vi "LED matrix.vi"() -> ()   [LabVIEW 2010]
uses:
  <vilib>/MakerHub/LINX/LMH-LINX.lvlib
  <vilib>/MakerHub/LINX/Private/Type Defs/Peripherals/SPI/SPI CS Logic Level.ctl
  <vilib>/MakerHub/LINX/Public/Peripherals/SPI/SPI CS Config.ctl
  <vilib>/MakerHub/LINX/Public/Peripherals/SPI/SPI Write Read N Frames.vi
  <vilib>/MakerHub/LINX/Private/Type Defs/Peripherals/SPI/SPI Bit Order.ctl
  <vilib>/MakerHub/LINX/Private/Type Defs/Peripherals/SPI/SPI Mode.ctl
  <vilib>/MakerHub/LINX/Private/Type Defs/Peripherals/SPI/SPI Configuration.ctl
  <vilib>/MakerHub/LINX/Public/Utilities/Open Serial.vi
panel:
  out "Title":string="LabVIEW Arduino and LED matrix"
  in  "4":bool[][](array[boolean])=[[TRUE, TRUE, TRUE, TRUE, TRUE, TRUE, TRUE, TRUE], [TRUE, FALSE, FALSE, FALSE, FALSE, FALSE, FALSE, TRUE], [TRUE, FALSE, FALSE, FALSE, FALSE, FALSE, FALSE, TRUE], [TRUE, FALSE, FALSE, FALSE, FALSE, FALSE, FALSE, TRUE], [TRUE, FALSE, FALSE, FALSE, FALSE, FALSE, FALSE, TRUE], [TRUE, FALSE, FALSE, FALSE, FALSE, FALSE, FALSE, TRUE], [TRUE, FALSE, FALSE, FALSE, FALSE, FALSE, FALSE, TRUE], [TRUE, TRUE, TRUE, TRUE, TRUE, TRUE, TRUE, TRUE]]
  in  "milliseconds to wait":u32=1000
  in  "Debug":bool
  in  "1":bool[][](array[boolean])=[[FALSE, FALSE, FALSE, FALSE, FALSE, FALSE, FALSE, FALSE], [FALSE, FALSE, FALSE, FALSE, FALSE, FALSE, FALSE, FALSE], [FALSE, FALSE, FALSE, FALSE, FALSE, FALSE, FALSE, FALSE], [FALSE, FALSE, FALSE, TRUE, TRUE, FALSE, FALSE, FALSE], [FALSE, FALSE, FALSE, TRUE, TRUE, FALSE, FALSE, FALSE], [FALSE, FALSE, FALSE, FALSE, FALSE, FALSE, FALSE, FALSE], [FALSE, FALSE, FALSE, FALSE, FALSE, FALSE, FALSE, FALSE], [FALSE, FALSE, FALSE, FALSE, FALSE, FALSE, FALSE, FALSE]]
  in  "2":bool[][](array[boolean])=[[FALSE, FALSE, FALSE, FALSE, FALSE, FALSE, FALSE, FALSE], [FALSE, FALSE, FALSE, FALSE, FALSE, FALSE, FALSE, FALSE], [FALSE, FALSE, TRUE, TRUE, TRUE, TRUE, FALSE, FALSE], [FALSE, FALSE, TRUE, FALSE, FALSE, TRUE, FALSE, FALSE], [FALSE, FALSE, TRUE, FALSE, FALSE, TRUE, FALSE, FALSE], [FALSE, FALSE, TRUE, TRUE, TRUE, TRUE, FALSE, FALSE], [FALSE, FALSE, FALSE, FALSE, FALSE, FALSE, FALSE, FALSE], [FALSE, FALSE, FALSE, FALSE, FALSE, FALSE, FALSE, FALSE]]
  in  "3":bool[][](array[boolean])=[[FALSE, FALSE, FALSE, FALSE, FALSE, FALSE, FALSE, FALSE], [FALSE, TRUE, TRUE, TRUE, TRUE, TRUE, TRUE, FALSE], [FALSE, TRUE, FALSE, FALSE, FALSE, FALSE, TRUE, FALSE], [FALSE, TRUE, FALSE, FALSE, FALSE, FALSE, TRUE, FALSE], [FALSE, TRUE, FALSE, FALSE, FALSE, FALSE, TRUE, FALSE], [FALSE, TRUE, FALSE, FALSE, FALSE, FALSE, TRUE, FALSE], [FALSE, TRUE, TRUE, TRUE, TRUE, TRUE, TRUE, FALSE], [FALSE, FALSE, FALSE, FALSE, FALSE, FALSE, FALSE, FALSE]]
  out "Loop":i32=8
  in  "Serial Port":refnum<visa-resource-name>="COM4"
  in  "SPI Frame Size":u8=2
  in  "SPI Channel (0)":u8
  in  "stop":bool
  # "Ricky"
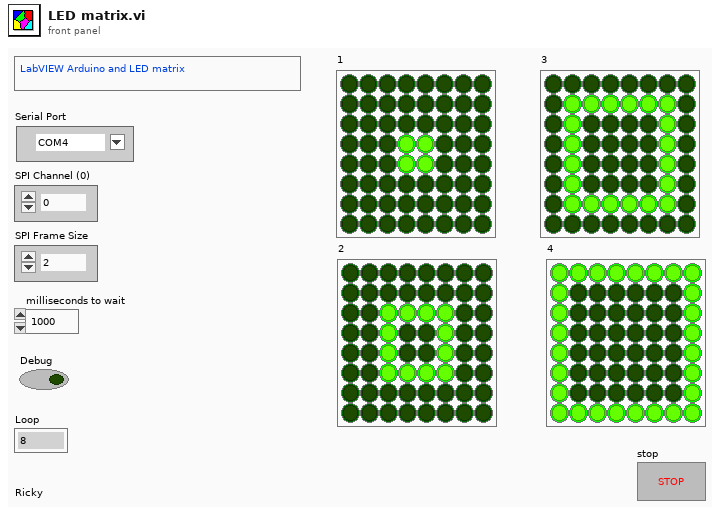
[diagram p1: front panel]
types:
  T1 = typedef "LMH-LINX.lvlib/SPI Configuration.ctl" = cluster{"Clock Frequency":u32, "Bit Order":T2, "SPI Mode":T3}
  T2 = typedef "LMH-LINX.lvlib/SPI Bit Order.ctl" = enum8{"LSb First", "MSb First"}
  T3 = typedef "LMH-LINX.lvlib/SPI Mode.ctl" = enum8{"Mode 0", "Mode 1", "Mode 2", "Mode 3"}
  T4 = typedef "LMH-LINX.lvlib/SPI CS Config.ctl" = cluster{"CS Channel":u8, "CS Logic Level":T5}
  T5 = typedef "LMH-LINX.lvlib/SPI CS Logic Level.ctl" = enum8{"Active Low", "Active High"}
  T6 = typedef "LMH-LINX.lvlib/LINX Ref.ctl" = cluster{"IO":T7, "Interface":T8, "LINX Device Config":T9}
  T7 = typedef "LMH-LINX.lvlib/Platform.ctl" = enum16{"Remote", "Local"}
  T8 = typedef "LMH-LINX.lvlib/Interface.ctl" = enum16{"Serial", "TCP"}
  T9 = typedef "LMH-LINX.lvlib/Device.lvlib/LINX Device Config.ctl" = cluster{"Interface":T8, "COM Port":refnum<visa-resource-name>, "TCP Configuration":T10, "Device Family":u8, "Device ID":u8, "Device Name":string, "TCP Ref":refnum<k5>, "Channels":T11}
  T10 = typedef "LMH-LINX.lvlib/Device.lvlib/TCP Config.ctl" = cluster{"IP Address":string, "Port":u16}
  T11 = typedef "LMH-LINX.lvlib/Channels.ctl" = cluster{"DI":u8[], "DO":u8[], "AI":u8[], "AO":u8[], "PWM":u8[], "QE":u8[], "UART":u8[], "I2C 2":u8[], "SPI":u8[], "CAN":u8[], "Servo":u8[], "AI Ref (V)":dbl, "AI Resolution (Bits)":u8, "AO Ref (V)":dbl, "AO Resolution (Bits)":u8}
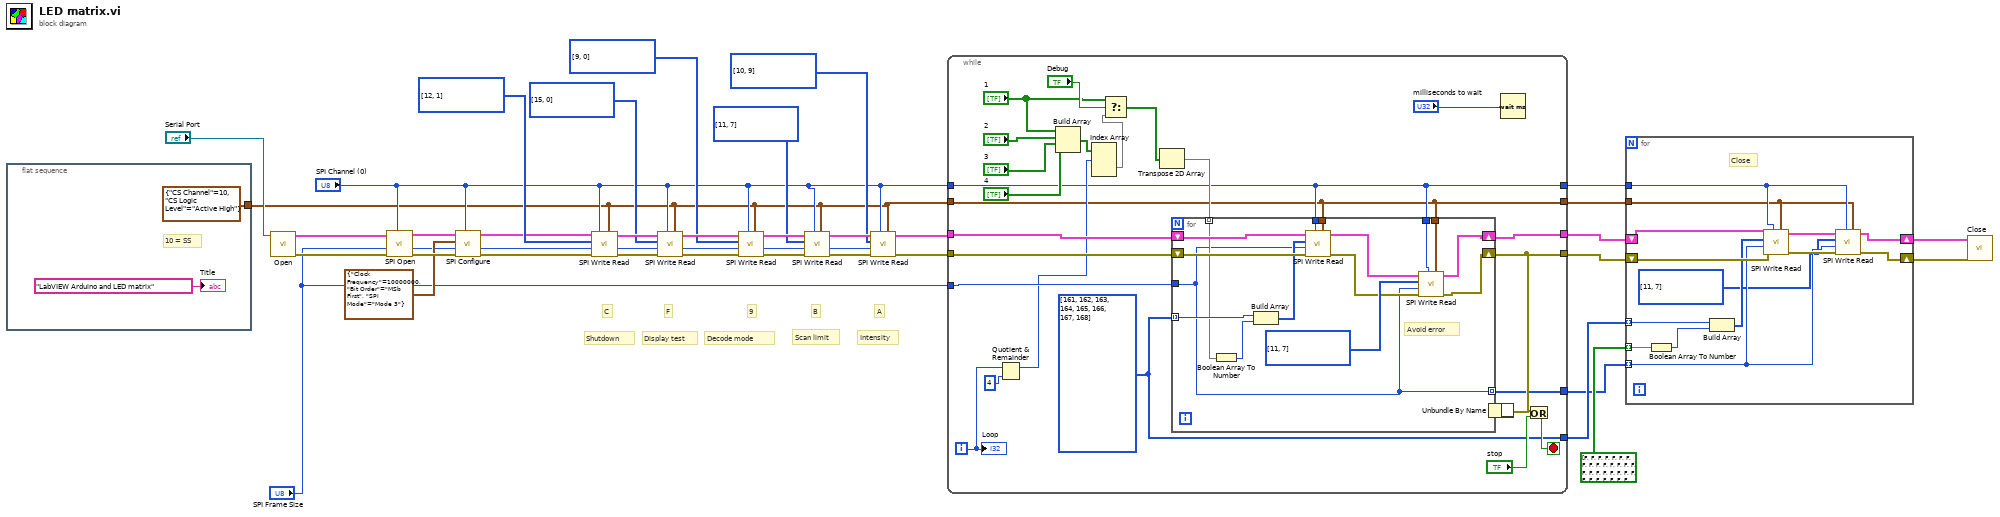
[diagram p0: block diagram]
diagram:
  # "Intensity"
  # "Decode mode"
  # "Display test"
  # "Shutdown"
  # "Scan limit"
  # "A"
  # "B"
  # "9"
  # "F"
  # "C"
  n1 = flat-sequence {
    tunnel: [T4 {"CS Channel"=10, "CS Logic Level"=enum."Active High"} ("CS Configuration")] -> w12
    frame #0 {
      # "10 = SS"
      "Title" <- "LabVIEW Arduino and LED matrix" ("Title")
    }
  }
  n2 = call-poly <vilib>:"Open.vi"("Serial Port"="Serial Port") -> ("Error Out"=w14:errorcluster, "LINX Resource"=w15:T6)  [unwired: 8 in, 1 out]
  n3 = call <vilib>:"SPI Open.vi"("SPI Channel (0)"="SPI Channel (0)", "Error In"=w14, "LINX Resource"=w15) -> ("Error Out"=w35:errorcluster, "LINX Resource"=w34:T6)  [unwired: 7 in]
  n4 = call <vilib>:"SPI Configure.vi"("SPI Channel (0)"="SPI Channel (0)", "Error In"=w35, "SPI Configuration"=T1 {"Clock Frequency"=10000000, "Bit Order"=enum."MSb First", "SPI Mode"=enum."Mode 3"}, "LINX Resource"=w34) -> ("Error Out"=w16:errorcluster, "LINX Resource"=w11:T6)  [unwired: 5 in, 1 out]
  n5 = call-poly <vilib>:"SPI Write Read.vi"("CS Configuration"=w12, "SPI Channel (0)"="SPI Channel (0)", "Error In"=w16, "SPI Frame Size"="SPI Frame Size", "Data"=u8[] [12, 1], "LINX Resource"=w11) -> ("Error Out"=w25:errorcluster, "LINX Resource"=w30:T6)  [unwired: 3 in, 1 out]
  n6 = call-poly <vilib>:"SPI Write Read.vi"("CS Configuration"=w12, "SPI Channel (0)"="SPI Channel (0)", "Error In"=w25, "SPI Frame Size"="SPI Frame Size", "Data"=u8[] [15, 0], "LINX Resource"=w30) -> ("Error Out"=w24:errorcluster, "LINX Resource"=w29:T6)  [unwired: 3 in, 1 out]
  n7 = call-poly <vilib>:"SPI Write Read.vi"("CS Configuration"=w12, "SPI Channel (0)"="SPI Channel (0)", "Error In"=w24, "SPI Frame Size"="SPI Frame Size", "Data"=u8[] [9, 0], "LINX Resource"=w29) -> ("Error Out"=w23:errorcluster, "LINX Resource"=w28:T6)  [unwired: 3 in, 1 out]
  n8 = call-poly <vilib>:"SPI Write Read.vi"("CS Configuration"=w12, "SPI Channel (0)"="SPI Channel (0)", "Error In"=w23, "SPI Frame Size"="SPI Frame Size", "Data"=u8[] [11, 7], "LINX Resource"=w28) -> ("Error Out"=w22:errorcluster, "LINX Resource"=w27:T6)  [unwired: 3 in, 1 out]
  n9 = call-poly <vilib>:"SPI Write Read.vi"("CS Configuration"=w12, "SPI Channel (0)"="SPI Channel (0)", "Error In"=w22, "SPI Frame Size"="SPI Frame Size", "Data"=u8[] [10, 9], "LINX Resource"=w27) -> ("Error Out"=w21:errorcluster, "LINX Resource"=w26:T6)  [unwired: 3 in, 1 out]
  n10 = while {
    tunnel: w26 -> [w61]
    tunnel: w21 -> [w59]
    tunnel: "SPI Channel (0)" -> [w42]
    tunnel: "SPI Frame Size" -> [w62]
    tunnel: [w60] -> w9
    tunnel: [w57] -> w8
    tunnel: w12 -> [w41]
    tunnel: [w42] -> w5
    tunnel: [w41] -> w4
    tunnel: [w40] -> w2
    tunnel: [w39] -> w1
    i -> [w51]
    stop <- w56 stop-if-true
    w40 = u8[] [161, 162, 163, 164, 165, 166, 167, 168]
    n11 = Quotient & Remainder(x=w51, y=4) -> (x-y*floor(x/y)=w49:i32)  [unwired: 1 out]
    n12 = Build Array("1", "2", "3", "4") -> (w52:bool[][][])
    n13 = Index Array(array=w52, index (dim 0)=w49) -> (element=w48:bool[][])  [unwired: 2 in]
    n14 = Select(t="1", s="Debug", f=w48) -> (s? t:f=w44:bool[][])
    n15 = Transpose 2D Array(2D array=w44) -> (transposed array=w55:bool[][])
    n16 = for {
      tunnel: w42 -> [w78]
      tunnel: w41 -> [w77]
      tunnel: w62 -> [w63]
      shift-right: [w69] -> w60
      shift-left: w61 -> [w76]
      shift-right: [w64] -> w57
      shift-left: w59 -> [w75]
      tunnel: w40 -> [w74] mode=indexing
      tunnel: w55 -> [w71] mode=indexing
      tunnel: w41 -> [w68]
      tunnel: w42 -> [w67]
      tunnel: [w63] -> w39 mode=indexing
      # "Avoid error"
      n17 = Boolean Array To Number(Boolean array=w71) -> (number=w72:u32)
      n18 = Build Array(w74, w72) -> (w73:u32[])
      n19 = call-poly <vilib>:"SPI Write Read.vi"("CS Configuration"=w77, "SPI Channel (0)"=w78, "Error In"=w75, "SPI Frame Size"=w63, "Data"=w73, "LINX Resource"=w76) -> ("Error Out"=w65:errorcluster, "LINX Resource"=w70:T6)  [unwired: 3 in, 1 out]
      n20 = call-poly <vilib>:"SPI Write Read.vi"("CS Configuration"=w68, "SPI Channel (0)"=w67, "Error In"=w65, "SPI Frame Size"=w63, "Data"=u8[] [11, 7], "LINX Resource"=w70) -> ("Error Out"=w64:errorcluster, "LINX Resource"=w69:T6)  [unwired: 3 in, 1 out]
    }
    n21 = Wait (ms)(milliseconds to wait="milliseconds to wait") -> ()  [unwired: 1 out]
    n22 = Or(y="stop") -> (x=w38:errorcluster, x .or. y?=w56:bool)
    n23 = Unbundle By Name(w57, w38) -> ()
    "Loop" <- w51
  }
  n24 = for {
    tunnel: w5 -> [w82]
    tunnel: w4 -> [w81]
    shift-right: [w85] -> w6
    shift-left: w9 -> [w92]
    shift-right: [w84] -> w7
    shift-left: w8 -> [w91]
    tunnel: bool[][] [[FALSE, FALSE, FALSE, FALSE, FALSE, FALSE, FALSE, FALSE], [FALSE, FALSE, FALSE, FALSE, FALSE, FALSE, FALSE, FALSE], [FALSE, FALSE, FALSE, FALSE, FALSE, FALSE, FALSE, FALSE], [FALSE, FALSE, FALSE, FALSE, FALSE, FALSE, FALSE, FALSE], [FALSE, FALSE, FALSE, FALSE, FALSE, FALSE, FALSE, FALSE], [FALSE, FALSE, FALSE, FALSE, FALSE, FALSE, FALSE, FALSE], [FALSE, FALSE, FALSE, FALSE, FALSE, FALSE, FALSE, FALSE], [FALSE, FALSE, FALSE, FALSE, FALSE, FALSE, FALSE, FALSE]] ("1") -> [w89] mode=indexing
    tunnel: w2 -> [w88] mode=indexing
    tunnel: w1 -> [w80] mode=indexing
    # "Close"
    n25 = Boolean Array To Number(Boolean array=w89) -> (number=w90:u32)
    n26 = Build Array(w88, w90) -> (w87:u32[])
    n27 = call-poly <vilib>:"SPI Write Read.vi"("CS Configuration"=w81, "SPI Channel (0)"=w82, "Error In"=w91, "SPI Frame Size"=w80, "Data"=w87, "LINX Resource"=w92) -> ("Error Out"=w83:errorcluster, "LINX Resource"=w86:T6)  [unwired: 3 in, 1 out]
    n28 = call-poly <vilib>:"SPI Write Read.vi"("CS Configuration"=w81, "SPI Channel (0)"=w82, "Error In"=w83, "SPI Frame Size"=w80, "Data"=u8[] [11, 7], "LINX Resource"=w86) -> ("Error Out"=w84:errorcluster, "LINX Resource"=w85:T6)  [unwired: 3 in, 1 out]
  }
  n29 = call <vilib>:"Close.vi"("Error In"=w7, "LINX Resource"=w6) -> ()  [unwired: 9 in, 1 out]
